vi "(Un)cover stop button.vi"(8 "error in (no error)":errorcluster, 9 "Cover/Uncover":bool, 10 "GUI ref in":refnum<vi>, 11 "Common GUI v3 in":refnum<class "Common GUI v3.lvclass">) -> (0 "error out":errorcluster, 2 "GUI ref out":refnum<vi>, 3 "Common GUI v3 out":refnum<class "Common GUI v3.lvclass">)   [LabVIEW 2026, in "TALOS.lvlib" / "Common GUI v3.lvlib" / "Common GUI v3.lvclass"]
uses:
  Common GUI v3.lvclass
  Ancestor/Ancestor/Ancestor.lvclass/Ancestor.ctl
  Support VIs/Generate Error.vi
  FGV/Error Memory/Get Error Description.vi
  Support VIs/Get PC name.vi
  Ancestor/Ancestor/Read ID.vi
  Support VIs/Get Class Name.vi
  <vilib>/Utility/error.llb/Clear Errors.vi
  FGV/Error Memory/Error Memory Core.vi
  <vilib>/AdvancedString/Delimited String to 1D String Array.vi
  <vilib>/AdvancedString/Delimited String to 1D String Array (string).vi
  Support VIs/Circus Root Path.vi
  FGV/Error Memory/Error Crt Lvl checker.vi
  FGV/Error Memory/Error Memory Core.vi/40c8088d-b597-4017-91af-faa98e00292e.vi
  FGV/Error Memory/Error Memory Core.vi/d4a3ab98-063c-4e44-b43d-fbdcfe6c2be2.vi
  Support VIs/Global Memory.vi
  <vilib>/Utility/LVClass/Get LV Class Name.vi
  Support VIs/Is in Packed Library.vi
  Support VIs/TALOS Root path.vi
  Support VIs/Read CSV worksheet.vi
  Support VIs/Global Constants.vi
  <vilib>/Utility/error.llb/General Error Handler.vi
  Support VIs/Error Log.vi
  Ancestor/Ancestor/Ancestor.lvclass
  <vilib>/Comparison/Equal/Equal Functor/Equal Functor.lvclass
  TALOS.lvlib
panel:
  in  "Closed Cover":refnum<vi>
  in  "Opened Cover":refnum<vi>
  # "These two controls are used as memory"
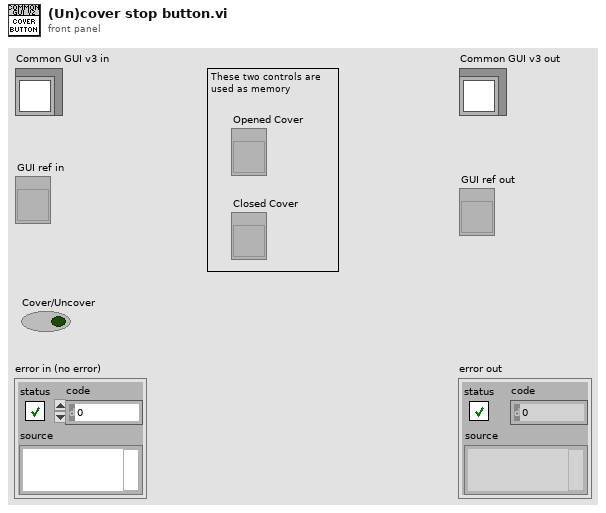
[diagram p1: front panel]
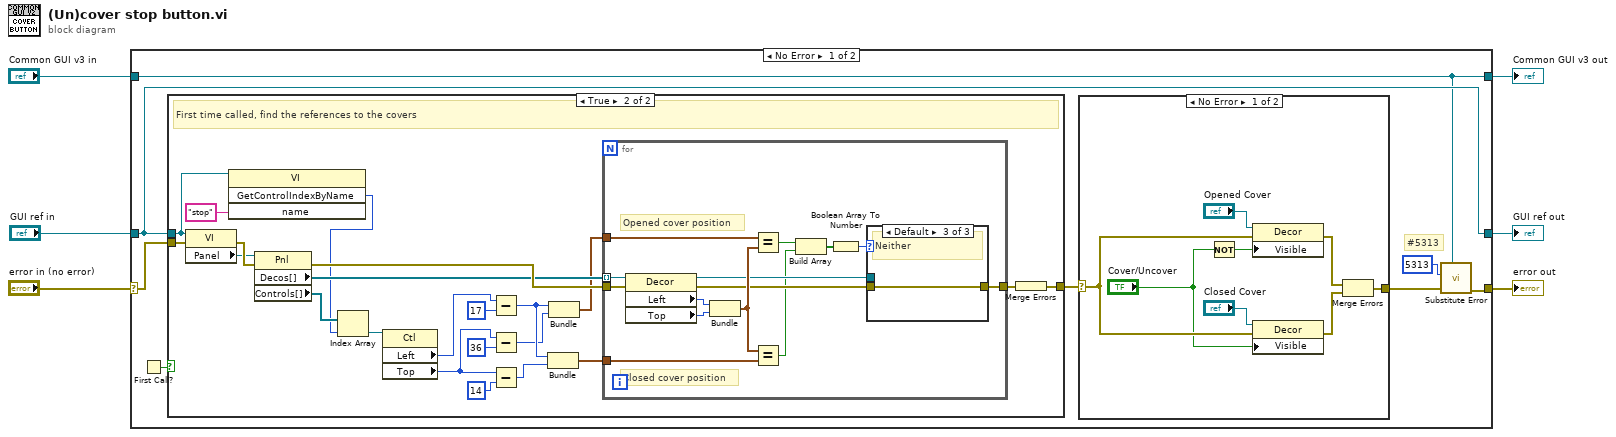
[diagram p0: block diagram]
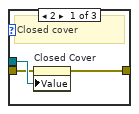
[diagram p3: hidden frame]
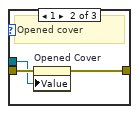
[diagram p4: hidden frame]
diagram:
  n1 = case shown="No Error" "error in (no error)" {
    selector: "error in (no error)" -> [w13 w70]
    tunnel: [w9 w70] -> w5
    tunnel: [w8 w69] -> w3
    tunnel: "Common GUI v3 in" -> [w8 w69]
    tunnel: "GUI ref in" -> [w12 w68]
    tunnel: [w12 w68] -> w1
    frame No Error {
      # "#5313"
      n2 = First Call?() -> (First Call?: T/F=w14:bool)
      n3 = case shown="True" w14 {
        tunnel: [w15 w31] -> w11
        tunnel: w12 -> [_ w20]
        tunnel: w13 -> [w15 w34]
        frame False {
          # "References should be saved, do nothing"
        }
        frame True {
          # "First time called, find the references to the covers"
          n4 = property class="VI"(reference=w20, error in=w34) -> (error out=w37:errorcluster, "Panel"=w35:refnum<vi>)  [unwired: 1 out]
          n5 = invoke class="VI" method="GetControlIndexByName"(reference=w20, "name"="stop" ("Control Name")) -> ("GetControlIndexByName"=w16:i32)  [unwired: 2 in, 3 out]
          n6 = property class="Pnl"(reference=w35, error in=w37) -> (error out=w33:errorcluster, "Decos[]"=w32:refnum<vi>[], "Controls[]"=w17:refnum<vi>[])  [unwired: 1 out]
          n7 = Index Array(array=w17, index=w16) -> (element=w18:refnum<vi>)
          n8 = property class="Ctl"(reference=w18) -> ("Left"=w28:i32, "Top"=w26:i32)  [unwired: 1 in, 2 out]
          n9 = Subtract(x=w28, y=17) -> (x-y=w27:i32)
          n10 = Subtract(x=w26, y=36) -> (x-y=w23:i32)
          n11 = Subtract(x=w26, y=14) -> (x-y=w24:i32)
          n12 = Bundle(w27, w24) -> (w21:cluster{i32, i32})  [unwired: 1 in]
          n13 = Bundle(w27, w23) -> (w22:cluster{i32, i32})  [unwired: 1 in]
          n14 = for {
            tunnel: w32 -> [w51] mode=indexing
            tunnel: w33 -> [w46]
            tunnel: [w44] -> w36
            tunnel: w22 -> [w42]
            tunnel: w21 -> [w43]
            # "Opened cover position"
            # "Closed cover position"
            n15 = property class="Decor"(reference=w51, error in=w46) -> (reference out=w47:refnum<vi>, error out=w45:errorcluster, "Left"=w50:i32, "Top"=w49:i32)
            n16 = Bundle("Left"=w50, "Top"=w49) -> (w48:cluster{"Left":i32, "Top":i32})  [unwired: 1 in]
            n17 = Equal?(x=w42, y=w48) -> (x = y?=w41:bool)
            n18 = Equal?(x=w48, y=w43) -> (x = y?=w40:bool)
            n19 = Build Array(w41, w40) -> (w39:bool[])
            n20 = Boolean Array To Number(Boolean array=w39) -> (number=w38:u32)
            n21 = case shown="Default" w38 {
              tunnel: w47 -> [w54 w55 _]
              tunnel: w45 -> [w53 w57 w58]
              tunnel: [w52 w56 w58] -> w44
              frame 2 {
                # "Closed cover"
                n22 = property on="Closed Cover" class="LVObjRef (strict)"(error in=w53, "Value"=w54) -> (error out=w52:errorcluster)  [unwired: 1 in, 1 out]
              }
              frame 1 {
                # "Opened cover"
                n23 = property on="Opened Cover" class="LVObjRef (strict)"(error in=w57, "Value"=w55) -> (error out=w56:errorcluster)  [unwired: 1 in, 1 out]
              }
              frame Default {
                # "Neither"
              }
            }
          }
          n24 = Merge Errors(w36) -> (w31:errorcluster)
        }
      }
      n25 = case shown="No Error" w11 {
        selector: w11 -> [w66 w67]
        tunnel: [w59 w67] -> w10
        frame No Error {
          n26 = Not(x="Cover/Uncover") -> (.not. x?=w61:bool)
          n27 = property class="Decor"(reference="Opened Cover", error in=w66, "Visible"=w61) -> (error out=w63:errorcluster)  [unwired: 1 out]
          n28 = property class="Decor"(reference="Closed Cover", error in=w66, "Visible"="Cover/Uncover") -> (error out=w62:errorcluster)  [unwired: 1 out]
          n29 = Merge Errors(w63, w62) -> (w59:errorcluster)
        }
        frame Error {
        }
      }
      n30 = call "Substitute Error.vi"("LabVIEW Object"=w8, "error in (no error)"=w10, "Error Code"=5313) -> ("error out"=w9:errorcluster)  [unwired: 8 in]
    }
    frame Error {
    }
  }
  "error out" <- w5
  "Common GUI v3 out" <- w3
  "GUI ref out" <- w1
